vi "structure.vi"() -> ()   [LabVIEW 2018]
panel:
  in  "左移与右移":bool
  in  "手动模式":bool
  in  "扫描开关":bool
  out "扫描结果":cluster{i32, dbl}[](graph)
  out "平均值":dbl
  out "传感器端口ai0":dynamicdata(graph)
  out "计次":dbl
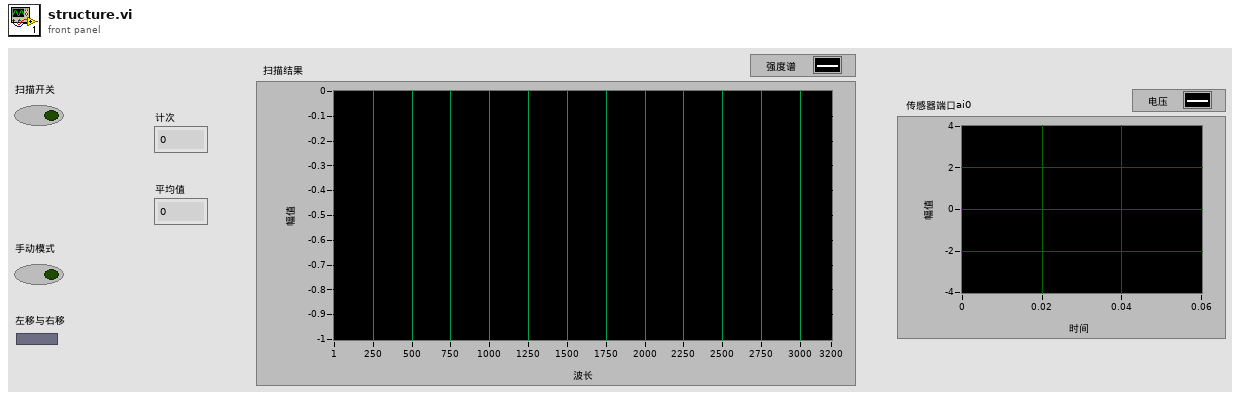
[diagram p1: front panel]
types:
  T1 = enum16{"open", "replace", "create", "open or create", "replace or create", "replace or create with confirmation"}
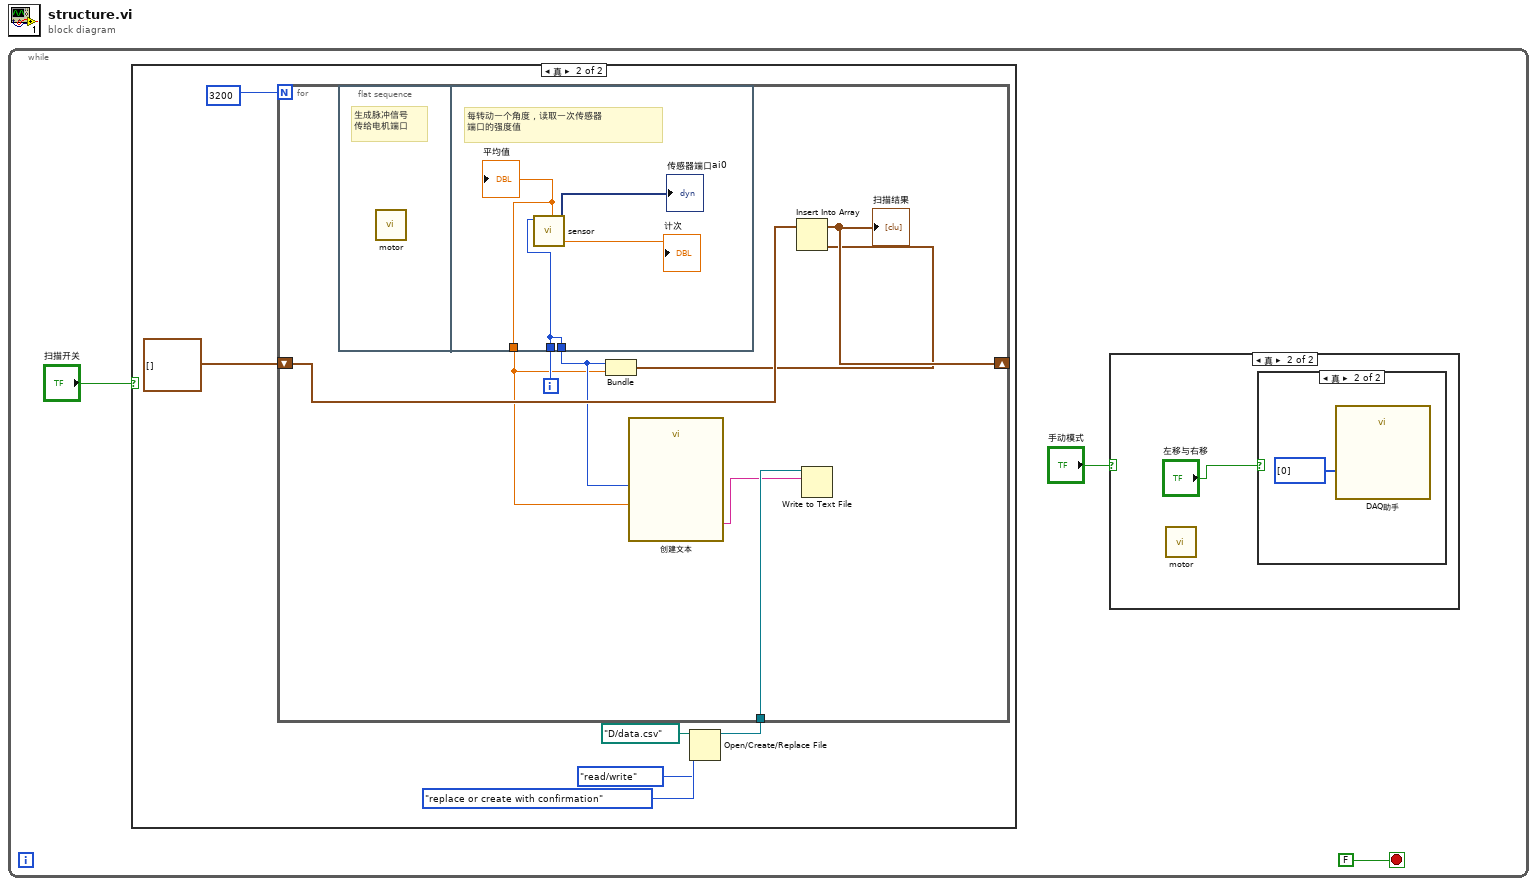
[diagram p0: block diagram]
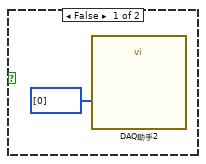
[diagram p3: hidden frame]
diagram:
  n1 = while {
    stop <- FALSE stop-if-true
    n2 = case shown="真" "扫描开关" {
      frame False {
      }
      frame True {
        n3 = Open/Create/Replace File(file path (use dialog)=path "D:/data.csv" ("文件路径（使用对话框）"), operation (0:open)=T1."replace or create with confirmation" ("操作(0:open)"), access (0:read/write)=enum16{"read/write", "read-only", "write-only"}."read/write" ("权限(0:read/write)")) -> (refnum out=w8:refnum<file>)  [unwired: 3 in, 2 out]
        n4 = for {
          N: 3200 -> [_]
          shift-right: [w18] -> _
          shift-left: cluster{i32, dbl}[] [] -> [w19]
          tunnel: w8 -> [w14]
          i -> [w20]
          n5 = flat-sequence {
            tunnel: w20 -> [w21]
            tunnel: [w22] -> w15
            tunnel: [w21] -> w16
            frame #0 {
              # "生成脉冲信号\n传给电机端口"
              n6 = call "motor.vi"() -> ()  [unwired: 12 in]
            }
            frame #1 {
              # "每转动一个角度，读取一次传感器\n端口的强度值"
              n7 = call "sensor.vi"("计次读取"=w21) -> ("计次输出"=→"计次":dbl, "传感器端口"=→"传感器端口ai0":dynamicdata, "传感器端口平均值"=w22:dbl)  [unwired: 8 in]
              "平均值" <- w22
            }
          }
          n8 = Bundle(w16, "传感器端口平均值"=w15) -> (w17:cluster{i32, "传感器端口平均值":dbl})  [unwired: 1 in]
          n9 = call "创建文本"("d"=w16, "f"=w15) -> ("Result"=w13:string)  [unwired: 12 in, 1 out]
          n10 = Insert Into Array(array=w19, new element=w17) -> (w18:cluster{i32, dbl}[])  [unwired: 1 in]
          "扫描结果" <- w18
          n11 = Write to Text File(file (use dialog)=w14, text=w13) -> ()  [unwired: 2 in, 3 out]
        }
      }
    }
    n12 = case shown="真" "手动模式" {
      frame False {
      }
      frame True {
        n13 = call "motor.vi"() -> ()  [unwired: 12 in]
        n14 = case shown="真" "左移与右移" {
          frame False {
            n15 = call "DAQ助手2"("data"=u32[] [0]) -> ()  [unwired: 17 in, 2 out]
          }
          frame True {
            n16 = call "DAQ助手"("data"=u32[] [0]) -> ()  [unwired: 17 in, 2 out]
          }
        }
      }
    }
  }
